vi "Nullable.vi"(11 "Type in":refnum<class "Type.lvclass">) -> (2 "Nullable":bool)   [LabVIEW 2020, in "Conditum.lvlib" / "Columns.lvlib" / "Type.lvclass"]
uses:
  Type.lvclass
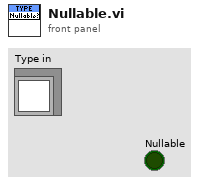
[diagram p1: front panel]
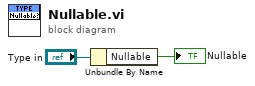
[diagram p0: block diagram]
diagram:
  n1 = Unbundle By Name("Type in") -> ("Nullable"=→"Nullable":bool)
